vi "Pockels Cal-AutoMeasure issue dialogue.vi"(9 "3 consecutive measurements are within +/-3mW of their previous one":bool, 10 "3 consecutive measurements are within +/-2mW":bool) -> (2 "Aborted by the user on detected issue":bool)   [LabVIEW 2017]
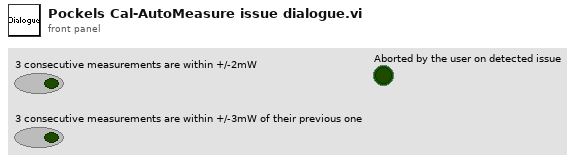
[diagram p1: front panel]
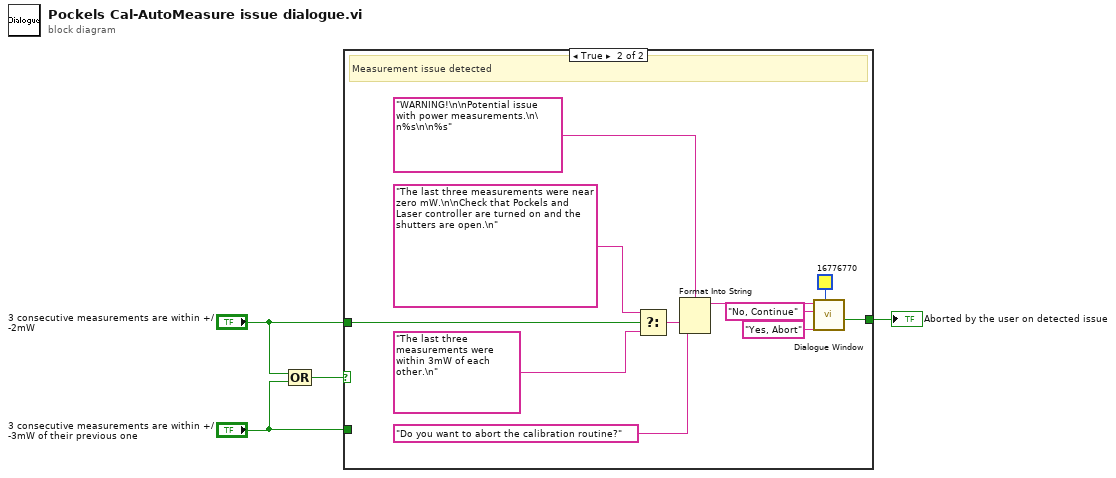
[diagram p0: block diagram]
diagram:
  n1 = Compound Arithmetic op=OR("3 consecutive measurements are within +/-2mW", "3 consecutive measurements are within +/-3mW of their previous one") -> (w2:bool)
  n2 = case shown="True" w2 {
    tunnel: "3 consecutive measurements are within +/-3mW of their previous one" -> [_ _]
    tunnel: "3 consecutive measurements are within +/-2mW" -> [_ w13]
    tunnel: [_ w6] -> w1
    frame False {
      # "No measurement issue"
    }
    frame True {
      # "Measurement issue detected"
      n3 = Select(t="The last three measurements were near zero mW.\n\nCheck that Pockels and Laser controller are turned on and the shutters are open.\n" ("Message string"), s=w13, f="The last three measurements were within 3mW of each other.\n" ("Message string")) -> (s? t:f=w10:string)
      n4 = Format Into String(format string="WARNING!\n\nPotential issue with power measurements.\n\n%s\n\n%s" ("Message string"), w10, "Do you want to abort the calibration routine?" ("input 2")) -> (resulting string=w9:string)  [unwired: 2 in, 1 out]
      n5 = call "Dialogue Window.vi"("Colour"=u32 16776770, "Caption-Left button (Cancel)"="Yes, Abort", "Caption-Right button (OK)"="No, Continue", "Message string"=w9) -> ("Cancelled (Left button pressed)"=w6:bool)  [unwired: 5 in, 2 out]
    }
  }
  "Aborted by the user on detected issue" <- w1
